vi "getInheritanceChain.vi"(8 "error in (no error)":errorcluster, 11 "Node in":refnum<class "Node.lvclass">) -> (0 "error out":errorcluster, 2 "Inheritance Chain":string[](array[string]), 3 "Node out":refnum<class "Node.lvclass">)   [LabVIEW 2009, in "Node.lvclass"]
doc: "Returns the inheritance chain."
uses:
  Node.lvclass
  DataObj/DataObj.lvclass
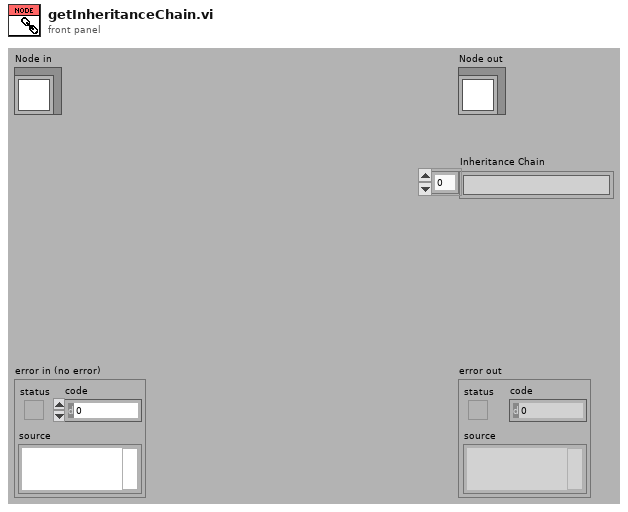
[diagram p1: front panel]
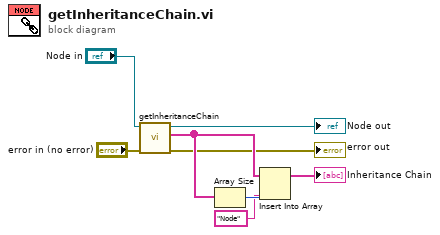
[diagram p0: block diagram]
diagram:
  n1 = call-parent "getInheritanceChain.vi"("error in (no error)"="error in (no error)", "DataObj in"="Node in") -> ("error out"=→"error out":errorcluster, "Inheritance Chain"=w5:string[], "DataObj out"=→"Node out":refnum<class "Node.lvclass">)  [unwired: 7 in]
  n2 = Array Size(array=w5) -> (size(s)=w6:i32)
  n3 = Insert Into Array(array=w5, index=w6, new element="Node") -> (→"Inheritance Chain":string[])
